vi "HFRR ADV v021 new software.vi"() -> ()   [LabVIEW 2025] (continued)
                    n2470 = Build Path(base path=w3624, name or relative path=w3626) -> (appended path=w3622:path)
                    n2471 = Number To Fractional String(number=w3652, width (-)=i16 5, precision (6)=i16 2) -> (F-format string=w3660:string)  [unwired: 1 in]
                    n2472 = local read "Fuel Discription :"() -> (w3648:string)
                    n2473 = local read "Batch Ref Num :"() -> (w3636:string)
                    n2474 = Get Date/Time String(date format (0)=enum16{"short", "long", "abbreviated"}."short") -> (date string=w3671:string, time string=w3668:string)  [unwired: 2 in]
                    n2475 = local read "Remarks :"() -> (w3647:string)
                    n2476 = Concatenate Strings("Load :- " ("Substring"), w3660, " grams ," ("Substring")) -> (w3659:string)
                    n2477 = local read "String 41"() -> (w3639:string)
                    n2478 = Concatenate Strings(w3648) -> (w3649:string)
                    n2479 = Concatenate Strings(w3636) -> (w3635:string)
                    n2480 = Concatenate Strings("tested by") -> (w3643:string)
                    n2481 = Concatenate Strings("(" ("Substring"), w3671, ")" ("Substring"), w3668) -> (w3641:string)
                    "concatenated string" <- w3641
                    n2482 = Concatenate Strings(w3647, "," ("string")) -> (w3646:string)
                    n2483 = Concatenate Strings("  TIME;      COF;       STROKE;     AIR TEMP;  TEMP;  HUMIDITY;  ECR; PID-OUT; FREQUENCY" ("Substring"), "\r") -> (w3655:string)
                    n2484 = Concatenate Strings(w3639, w3638, "Fuel Discription :-" ("Substring"), w3649, w3638, w3659, w3638, "Batch Ref Num :-" ("Substring"), w3635, w3638, " Remarks :- " ("Substring"), w3646, w3638, " Date :- " ("Substring"), w3641, w3638, "Tested By :-" ("Substring"), w3643) -> (w3653:string)
                    "REMARKS" <- w3653
                    n2485 = call <vilib>:"Write Characters To File.vi"("append to file? (new file:F)"=FALSE, "character string"=w3655, "file path (dialog if empty)"=w3623) -> ()  [unwired: 2 in, 1 out]
                    n2486 = call <vilib>:"Write Characters To File.vi"("append to file? (new file:F)"=FALSE, "character string"=w3653, "file path (dialog if empty)"=w3622) -> ()  [unwired: 2 in, 1 out]
                  }
                  frame #2 {
                    n2487 = local write "Cycles elapsed"(0 ("Cycles elapsed")) -> ()
                    n2488 = local write "cyclecount"(0 ("cyclecount")) -> ()
                    n2489 = local write "Save & Continue"(FALSE ("OK")) -> ()
                    n2490 = local write "autostrtflg"(TRUE ("autostrtflg")) -> ()
                    n2491 = local write "Save"(FALSE ("Save")) -> ()
                    n2492 = Get Date/Time In Seconds() -> (seconds since 1Jan1904=w3678:timestamp)
                    n2493 = To Double Precision Float(number=w3678) -> (double precision float=w3677:dbl)
                    n2494 = local write "acq timer"(w3677) -> ()
                    n2495 = One Button Dialog(message="Please ensure sample is mounted properly and machine is ready in all aspects for testing !", button name ("OK")="Ok") -> ()  [unwired: 1 out]
                  }
                  frame #3 {
                    n2496 = stacked-sequence {
                      frame #0 {
                        n2497 = local write "Main Dashboard Buttons"(T1."Dashboard" ("Main Dashboard Buttons")) -> ()
                        n2498 = local write "Main Tab"(T2."Acquire" ("Main Tab")) -> ()
                      }
                      frame #1 {
                        n2499 = local write "EVENT LOG"("" ("EVENT LOG")) -> ()
                      }
                      frame #2 {
                        n2500 = Wait (ms)(milliseconds to wait=u32 50) -> ()  [unwired: 1 out]
                      }
                      frame #3 {
                        n2501 = disable-structure shown="Disabled" {
                          frame Disabled {
                            n2502 = local read "EVENT LOG"() -> (w3690:string)
                            n2503 = call "Event Log.vi"("Content"="Test Details", "EVENT LOG"=w3690) -> ("EVENT LOG"=w3689:string)  [unwired: 8 in, 1 out]
                            n2504 = local write "EVENT LOG"(w3689) -> ()
                          }
                          frame Enabled {
                          }
                        }
                      }
                      frame #4 {
                        n2505 = Wait (ms)(milliseconds to wait=u32 50) -> ()  [unwired: 1 out]
                      }
                      frame #5 {
                        n2506 = local read "FILE"() -> (w3692:string)
                        n2507 = Concatenate Strings("File Name :" ("Content"), w3692) -> (w3693:string)
                        n2508 = local read "EVENT LOG"() -> (w3696:string)
                        n2509 = call "Event Log.vi"("Content"=w3693, "EVENT LOG"=w3696) -> ("EVENT LOG"=w3695:string)  [unwired: 8 in, 1 out]
                        n2510 = local write "EVENT LOG"(w3695) -> ()
                      }
                      frame #6 {
                        n2511 = Wait (ms)(milliseconds to wait=u32 50) -> ()  [unwired: 1 out]
                      }
                      frame #7 {
                        n2512 = local read "Batch Ref Num :"() -> (w3698:string)
                        n2513 = Concatenate Strings("Batch Ref No :" ("Content"), w3698) -> (w3699:string)
                        n2514 = local read "EVENT LOG"() -> (w3702:string)
                        n2515 = call "Event Log.vi"("Content"=w3699, "EVENT LOG"=w3702) -> ("EVENT LOG"=w3701:string)  [unwired: 8 in, 1 out]
                        n2516 = local write "EVENT LOG"(w3701) -> ()
                      }
                      frame #8 {
                        n2517 = Wait (ms)(milliseconds to wait=u32 50) -> ()  [unwired: 1 out]
                      }
                      frame #9 {
                        n2518 = local read "tested by"() -> (w3704:string)
                        n2519 = Concatenate Strings("Tested By :" ("Content"), w3704) -> (w3705:string)
                        n2520 = local read "EVENT LOG"() -> (w3708:string)
                        n2521 = call "Event Log.vi"("Content"=w3705, "EVENT LOG"=w3708) -> ("EVENT LOG"=w3707:string)  [unwired: 8 in, 1 out]
                        n2522 = local write "EVENT LOG"(w3707) -> ()
                      }
                      frame #10 {
                        n2523 = Wait (ms)(milliseconds to wait=u32 50) -> ()  [unwired: 1 out]
                      }
                      frame #11 {
                        n2524 = local read "TEST STANDARD"() -> (w3711:T3)
                        n2525 = case shown="\"ASTM D6079\", Default" w3711 {
                          tunnel: ["ASTM D6079" "ISO 12156" "CEC F-096-A-06" "Custom"] -> w3710
                          frame "ASTM D6079", Default {
                          }
                          frame "ISO 12156" {
                          }
                          frame "CEC F-096-A-06" {
                          }
                          frame "Custom" {
                          }
                        }
                        n2526 = Concatenate Strings("Test Standard :" ("Content"), w3710) -> (w3712:string)
                        n2527 = local read "EVENT LOG"() -> (w3715:string)
                        n2528 = call "Event Log.vi"("Content"=w3712, "EVENT LOG"=w3715) -> ("EVENT LOG"=w3714:string)  [unwired: 8 in, 1 out]
                        n2529 = local write "EVENT LOG"(w3714) -> ()
                      }
                      frame #12 {
                        n2530 = Wait (ms)(milliseconds to wait=u32 50) -> ()  [unwired: 1 out]
                      }
                      frame #13 {
                        n2531 = local read "Fuel Discription :"() -> (w3721:string)
                        n2532 = Concatenate Strings("Fuel Description :" ("Content"), w3721) -> (w3722:string)
                        n2533 = local read "EVENT LOG"() -> (w3725:string)
                        n2534 = call "Event Log.vi"("Content"=w3722, "EVENT LOG"=w3725) -> ("EVENT LOG"=w3724:string)  [unwired: 8 in, 1 out]
                        n2535 = local write "EVENT LOG"(w3724) -> ()
                      }
                      frame #14 {
                        n2536 = Wait (ms)(milliseconds to wait=u32 50) -> ()  [unwired: 1 out]
                      }
                      frame #15 {
                        n2537 = local read "Remarks :"() -> (w3727:string)
                        n2538 = Concatenate Strings("Remarks :" ("Content"), w3727) -> (w3728:string)
                        n2539 = local read "EVENT LOG"() -> (w3731:string)
                        n2540 = call "Event Log.vi"("Content"=w3728, "EVENT LOG"=w3731) -> ("EVENT LOG"=w3730:string)  [unwired: 8 in, 1 out]
                        n2541 = local write "EVENT LOG"(w3730) -> ()
                      }
                      frame #16 {
                        n2542 = Wait (ms)(milliseconds to wait=u32 50) -> ()  [unwired: 1 out]
                      }
                      frame #17 {
                        n2543 = local read "Operator ID"() -> (w3733:string)
                        n2544 = Concatenate Strings("Operator ID :" ("Content"), w3733) -> (w3735:string)
                        n2545 = local read "EVENT LOG"() -> (w3737:string)
                        n2546 = call "Event Log.vi"("Content"=w3735, "EVENT LOG"=w3737) -> ("EVENT LOG"=w3736:string)  [unwired: 8 in, 1 out]
                        n2547 = local write "EVENT LOG"(w3736) -> ()
                      }
                      frame #18 {
                        n2548 = Wait (ms)(milliseconds to wait=u32 50) -> ()  [unwired: 1 out]
                      }
                      frame #19 {
                        n2549 = disable-structure shown="Disabled" {
                          frame Disabled {
                            n2550 = local read "EVENT LOG"() -> (w3741:string)
                            n2551 = call "Event Log.vi"("Content"="Test Parameter", "EVENT LOG"=w3741) -> ("EVENT LOG"=w3740:string)  [unwired: 8 in, 1 out]
                            n2552 = local write "EVENT LOG"(w3740) -> ()
                          }
                          frame Enabled {
                          }
                        }
                      }
                      frame #20 {
                        n2553 = Wait (ms)(milliseconds to wait=u32 50) -> ()  [unwired: 1 out]
                      }
                      frame #21 {
                        n2554 = local read "Set Hz"() -> (w3745:dbl)
                        n2555 = Number To Fractional String(number=w3745, precision (6)=i16 2) -> (F-format string=w3744:string)  [unwired: 2 in]
                        n2556 = Concatenate Strings("Set Frequency [Hz] :" ("Content"), w3744) -> (w3747:string)
                        n2557 = local read "EVENT LOG"() -> (w3749:string)
                        n2558 = call "Event Log.vi"("Content"=w3747, "EVENT LOG"=w3749) -> ("EVENT LOG"=w3748:string)  [unwired: 8 in, 1 out]
                        n2559 = local write "EVENT LOG"(w3748) -> ()
                      }
                      frame #22 {
                        n2560 = Wait (ms)(milliseconds to wait=u32 50) -> ()  [unwired: 1 out]
                      }
                      frame #23 {
                        n2561 = local read "NORMAL LOAD"() -> (w3752:dbl)
                        n2562 = Number To Fractional String(number=w3752, precision (6)=i16 2) -> (F-format string=w3753:string)  [unwired: 2 in]
                        n2563 = Concatenate Strings("Applied Load [grams] :" ("Content"), w3753) -> (w3755:string)
                        n2564 = local read "EVENT LOG"() -> (w3757:string)
                        n2565 = call "Event Log.vi"("Content"=w3755, "EVENT LOG"=w3757) -> ("EVENT LOG"=w3756:string)  [unwired: 8 in, 1 out]
                        n2566 = local write "EVENT LOG"(w3756) -> ()
                      }
                      frame #24 {
                        n2567 = Wait (ms)(milliseconds to wait=u32 50) -> ()  [unwired: 1 out]
                      }
                      frame #25 {
                        n2568 = local read "Set Strk"() -> (w3760:dbl)
                        n2569 = Number To Fractional String(number=w3760, precision (6)=i16 2) -> (F-format string=w3761:string)  [unwired: 2 in]
                        n2570 = Concatenate Strings("Set Stroke [mm] :" ("Content"), w3761) -> (w3763:string)
                        n2571 = local read "EVENT LOG"() -> (w3765:string)
                        n2572 = call "Event Log.vi"("Content"=w3763, "EVENT LOG"=w3765) -> ("EVENT LOG"=w3764:string)  [unwired: 8 in, 1 out]
                        n2573 = local write "EVENT LOG"(w3764) -> ()
                      }
                      frame #26 {
                        n2574 = Wait (ms)(milliseconds to wait=u32 50) -> ()  [unwired: 1 out]
                      }
                      frame #27 {
                        n2575 = local read "Set Temp"() -> (w3768:dbl)
                        n2576 = Number To Fractional String(number=w3768, precision (6)=i16 2) -> (F-format string=w3769:string)  [unwired: 2 in]
                        n2577 = Concatenate Strings("Set Temperature [deg C] :" ("Content"), w3769) -> (w3771:string)
                        n2578 = local read "EVENT LOG"() -> (w3773:string)
                        n2579 = call "Event Log.vi"("Content"=w3771, "EVENT LOG"=w3773) -> ("EVENT LOG"=w3772:string)  [unwired: 8 in, 1 out]
                        n2580 = local write "EVENT LOG"(w3772) -> ()
                      }
                      frame #28 {
                        n2581 = Wait (ms)(milliseconds to wait=u32 50) -> ()  [unwired: 1 out]
                      }
                      frame #29 {
                        n2582 = local read "Set Rh"() -> (w3776:dbl)
                        n2583 = Number To Fractional String(number=w3776, precision (6)=i16 2) -> (F-format string=w3777:string)  [unwired: 2 in]
                        n2584 = Concatenate Strings("Set Humidity [%RH] :" ("Content"), w3777) -> (w3779:string)
                        n2585 = local read "EVENT LOG"() -> (w3781:string)
                        n2586 = call "Event Log.vi"("Content"=w3779, "EVENT LOG"=w3781) -> ("EVENT LOG"=w3780:string)  [unwired: 8 in, 1 out]
                        n2587 = local write "EVENT LOG"(w3780) -> ()
                      }
                      frame #30 {
                        n2588 = Wait (ms)(milliseconds to wait=u32 50) -> ()  [unwired: 1 out]
                      }
                      frame #31 {
                        n2589 = local read "test time"() -> (w3784:dbl)
                        n2590 = Number To Fractional String(number=w3784, precision (6)=i16 1) -> (F-format string=w3785:string)  [unwired: 2 in]
                        n2591 = Concatenate Strings("Test Duration [mins] :" ("Content"), w3785) -> (w3787:string)
                        n2592 = local read "EVENT LOG"() -> (w3789:string)
                        n2593 = call "Event Log.vi"("Content"=w3787, "EVENT LOG"=w3789) -> ("EVENT LOG"=w3788:string)  [unwired: 8 in, 1 out]
                        n2594 = local write "EVENT LOG"(w3788) -> ()
                      }
                      frame #32 {
                        w3790 = dbl[] [] ("History Data")
                        w3791 = cluster{"y":dbl, dbl, "y":dbl}[] [] ("History Data")
                        w3792 = FALSE ("Visible")
                        n2595 = property on="Stroke ( mm )" class="WFChart (strict)"("History Data"=w3791) -> ()  [unwired: 2 in, 2 out]
                        n2596 = property on="Humidity ( %RH )" class="WFChart (strict)"("History Data"=w3790) -> ()  [unwired: 2 in, 2 out]
                        n2597 = property on="Temperature ( Deg C )" class="WFChart (strict)"("History Data"=w3790) -> ()  [unwired: 2 in, 2 out]
                        n2598 = property on="Electrical Contact Resistance ( % )" class="WFChart (strict)"("History Data"=w3790) -> ()  [unwired: 2 in, 2 out]
                        n2599 = property on="Coefficient of Friction" class="WFChart (strict)"("History Data"=w3790) -> ()  [unwired: 2 in, 2 out]
                        n2600 = property on="Frictional Force ( N )" class="WFChart (strict)"("History Data"=w3790) -> ()  [unwired: 2 in, 2 out]
                        n2601 = property on="Coefficient of Friction" class="WFChart (strict)"("History Data"=w3790) -> ()  [unwired: 2 in, 2 out]
                        n2602 = property on="Frictional Force ( N )" class="WFChart (strict)"("History Data"=w3790) -> ()  [unwired: 2 in, 2 out]
                        n2603 = property on="Electrical Contact Resistance ( % )" class="WFChart (strict)"("History Data"=w3790) -> ()  [unwired: 2 in, 2 out]
                        n2604 = property on="Humidity ( %RH )" class="WFChart (strict)"("History Data"=w3790) -> ()  [unwired: 2 in, 2 out]
                        n2605 = property on="Stroke ( mm )" class="WFChart (strict)"("History Data"=w3791) -> ()  [unwired: 2 in, 2 out]
                        n2606 = property on="Temperature ( Deg C )" class="WFChart (strict)"("History Data"=w3790) -> ()  [unwired: 2 in, 2 out]
                        n2607 = property on="Service Password Log" class="Str"("Visible"=w3792) -> ()  [unwired: 2 in, 2 out]
                        n2608 = property on="Password 3" class="Clust (strict)"("Visible"=w3792) -> ()  [unwired: 2 in, 2 out]
                      }
                    }
                    "TEST FILE NAM,E SAVED" <- TRUE ("TEST FILE NAM,E SAVED")
                  }
                }
              }
            }
          }
        }
        n2609 = case shown="True" w3089 {
          frame False {
            n2610 = local write "tfalg"(0.0 ("tfalg")) -> ()
          }
          frame True {
            n2611 = local read "tfalg"() -> (w3234:dbl)
            n2612 = Equal?(x=w3234, y=0.0) -> (x = y?=w3235:bool)
            n2613 = case shown="True" w3235 {
              frame False {
              }
              frame True {
                n2614 = local read "Total No. of Tests"() -> (w3238:dbl)
                n2615 = local write "tfalg"(1.0 ("tfalg")) -> ()
                n2616 = local write "acq 2"(FALSE ("acq 2")) -> ()
                n2617 = Wait (ms)(milliseconds to wait=u32 200) -> ()  [unwired: 1 out]
                n2618 = Increment(x=w3238) -> (x+1=w3237:dbl)
                n2619 = local write "Total No. of Tests"(w3237) -> ()
              }
            }
          }
        }
        n2620 = local write "Test \nStatus"(w3095) -> ()
        n2621 = local write "Save"(w3095) -> ()
        n2622 = local read "Main Tab"() -> (w3052:T2)
        n2623 = case shown="True" w3076 {
          tunnel: [FALSE ("RUN") TRUE ("RUN")] -> w3075
          tunnel: [_ 1] -> w3068
          frame False {
          }
          frame True {
          }
        }
        n2624 = In Range and Coerce(upper limit=w3083, x=w3056, lower limit=w3082) -> (In Range?=w3074:bool)  [unwired: 1 out]
        n2625 = In Range and Coerce(upper limit=w3080, x=w3055, lower limit=w3081) -> (In Range?=w3072:bool)  [unwired: 1 out]
        n2626 = case shown="True" w3088 {
          frame False {
            n2627 = local read "Rt 3"() -> (w3216:bool)
            n2628 = case shown="True" w3216 {
              frame False {
              }
              frame True {
                n2629 = local write "Rt 3"(FALSE ("Rt 3")) -> ()
                n2630 = local write "Json End Flg"(TRUE ("Upld AR 2")) -> ()
              }
            }
            "Rt" <- TRUE ("Rt")
            "Rt 2" <- FALSE ("Rt")
          }
          frame True {
            n2631 = local read "Rt"() -> (w3223:bool)
            n2632 = local write "Rt 2"(TRUE ("Rt 2")) -> ()
            n2633 = case shown="True" w3223 {
              frame False {
              }
              frame True {
                w3224 = TRUE ("Upld AR 2")
                n2634 = local write "Rt"(FALSE ("Rt")) -> ()
                n2635 = local write "Upld AR"(w3224) -> ()
                n2636 = local write "Json St Flg"(w3224) -> ()
              }
            }
            "Rt 3" <- TRUE ("Rt 3")
          }
        }
        n2637 = case shown="True" w3074 {
          tunnel: [FALSE ("RUN") TRUE ("RUN")] -> w3073
          tunnel: [_ 2] -> w3067
          frame False {
          }
          frame True {
          }
        }
        n2638 = case shown="True" w3072 {
          tunnel: [FALSE ("RUN") TRUE ("RUN")] -> w3071
          tunnel: [_ 3] -> w3066
          frame False {
          }
          frame True {
          }
        }
        n2639 = case shown="\"Acquire\"" w3052 {
          tunnel: w3054 -> [_ w3285]
          frame Default {
            w3284 = 0.0 ("output")
            n2640 = local write "PID-out"(w3284) -> ()
            n2641 = local write "Frequency ( Hz )"(w3284) -> ()
          }
          frame "Acquire" {
            n2642 = stacked-sequence {
              frame #0 {
                n2643 = local read "Auto Start Test"() -> (w3287:bool)
                n2644 = case shown="True" w3287 {
                  tunnel: "RUN" -> [w3308 w3311]
                  tunnel: [w3308 w3310] -> w3288
                  frame False {
                  }
                  frame True {
                    n2645 = local read "Auto Start Temp"() -> (w3309:bool)
                    n2646 = Or(x=w3311, y=w3309) -> (x .or. y?=w3310:bool)
                  }
                }
                n2647 = local read "clk"() -> (w3307:dbl)
                n2648 = local read "Save"() -> (w3303:bool)
                n2649 = Equal?(x=w3307, y=0.0) -> (x = y?=w3304:bool)
                n2650 = And(x=w3304, y=w3303) -> (x .and. y?=w3305:bool)
                n2651 = Not(x="Engage") -> (.not. x?=w3294:bool)
                n2652 = case shown="False" w3288 {
                  tunnel: [0.0 w3334] -> w3290
                  frame False {
                    (unwired) TRUE ("Visible")
                    n2653 = local read "Auto Start Test"() -> (w3315:bool)
                    n2654 = local write "Start Time"(TRUE ("Start Time")) -> ()
                    n2655 = property on="Stroke 2" class="DigNum (strict)"("Visible"=FALSE) -> ()  [unwired: 2 in, 2 out]
                    n2656 = case shown="False" w3315 {
                      frame False {
                        n2657 = property on="Heater Button" class="Bool (strict)"("DisabledEnum"=T19."Enabled" ("Disabled")) -> ()  [unwired: 2 in, 2 out]
                        n2658 = property on="Humidity" class="Bool (strict)"("DisabledEnum"=T19."Enabled" ("Disabled")) -> ()  [unwired: 2 in, 2 out]
                      }
                      frame True {
                      }
                    }
                    n2659 = case shown="False" "TestCompFlg" {
                      frame False {
                        n2660 = local read "StartFlg"() -> (w3323:bool)
                        n2661 = case shown="True" w3323 {
                          frame False {
                          }
                          frame True {
                            n2662 = stacked-sequence {
                              frame #0 {
                                n2663 = local read "EVENT LOG"() -> (w3327:string)
                                n2664 = call "Event Log.vi"("Content"="Test was interrupted", "EVENT LOG"=w3327) -> ("EVENT LOG"=w3328:string)  [unwired: 8 in, 1 out]
                                n2665 = local write "EVENT LOG"(w3328) -> ()
                                n2666 = property on="RUN" class="Bool (strict)"("Visible"=TRUE) -> ()  [unwired: 2 in, 2 out]
                                n2667 = property on="Auto Start Test" class="Bool (strict)"("Visible"=TRUE) -> ()  [unwired: 2 in, 2 out]
                              }
                              frame #1 {
                                w3330 = FALSE ("StartFlg")
                                n2668 = property on="Heater Button" class="Bool (strict)"("Val(Sgnl)"=FALSE ("Value (Signaling)")) -> ()  [unwired: 2 in, 2 out]
                                n2669 = local write "Heater Button"(w3330) -> ()
                                n2670 = local write "StartFlg"(w3330) -> ()
                                n2671 = local write "Humidity"(w3330) -> ()
                              }
                              frame #2 {
                                n2672 = local write "Command"("VC;0" ("Command")) -> ()
                              }
                              frame #3 {
                                n2673 = Wait (ms)(milliseconds to wait=u32 1500) -> ()  [unwired: 1 out]
                              }
                              frame #4 {
                                n2674 = local write "Command"("HE;0" ("Command")) -> ()
                              }
                            }
                          }
                        }
                      }
                      frame True {
                      }
                    }
                    n2675 = local write "String 14"("Test will autostart once parameters reach the set value." ("String 14")) -> ()
                  }
                  frame True {
                    (unwired) FALSE ("Visible")
                    n2676 = property on="Stroke 2" class="DigNum (strict)"("Visible"=TRUE) -> ()  [unwired: 2 in, 2 out]
                    n2677 = property on="STOP 2" class="Bool (strict)"("Disabled"=u8 2) -> ()  [unwired: 2 in, 2 out]
                    n2678 = local write "String 14"(" Running....." ("String 14")) -> ()
                    n2679 = property on="Heater Button" class="Bool (strict)"("DisabledEnum"=T19."Disabled and Grayed Out" ("Disabled")) -> ()  [unwired: 2 in, 2 out]
                    n2680 = property on="Humidity" class="Bool (strict)"("DisabledEnum"=T19."Disabled and Grayed Out" ("Disabled")) -> ()  [unwired: 2 in, 2 out]
                    n2681 = case shown="True" "Start Time" {
                      selector: "Start Time" -> [_ w3353]
                      frame False {
                      }
                      frame True {
                        n2682 = Not(x=w3353) -> (.not. x?=w3352:bool)
                        n2683 = local write "Start Time"(w3352) -> ()
                        n2684 = local read "EVENT LOG"() -> (w3354:string)
                        n2685 = call "Event Log.vi"("Content"="Test in progress", "EVENT LOG"=w3354) -> ("EVENT LOG"=w3356:string)  [unwired: 8 in, 1 out]
                        n2686 = local write "EVENT LOG"(w3356) -> ()
                      }
                    }
                    n2687 = disable-structure shown="Enabled" {
                      disable-tunnel: [w3345 w3351] -> w3334
                      frame Disabled {
                        n2688 = local read "Set Hz"() -> (w3348:dbl)
                        n2689 = call <vilib>:"Uniform White Noise Waveform.vi"() -> ("signal out"=w3347:waveform(dbl))  [unwired: 10 in, 1 out]
                        n2690 = Random Number (0-1)() -> (number: 0 to 1=w3344:dbl)
                        n2691 = Add(x=w3348, y=w3347) -> (x+y=w3346:waveform(dbl))
                        n2692 = Multiply(x=ext 0.01 ("y"), y=w3344) -> (x*y=w3342:ext)
                        n2693 = Multiply(x=w3346, y=w3342) -> (x*y=w3345:waveform(ext))
                      }
                      frame Enabled {
                        n2694 = call-poly <vilib>:"Random Number (Range).vi"("lower bound (0)"=49.89, "upper bound (100)"=50.8) -> ("number"=w3351:dbl)  [unwired: 9 in]
                      }
                    }
                    "StartFlg" <- TRUE ("StartFlg")
                  }
                }
                n2695 = case shown="True" w3305 {
                  frame False {
                  }
                  frame True {
                    n2696 = local write "clk"(10.0 ("clk")) -> ()
                    n2697 = Get Date/Time In Seconds() -> (seconds since 1Jan1904=w3359:timestamp)
                    n2698 = To Double Precision Float(number=w3359) -> (double precision float=w3357:dbl)
                    n2699 = local write "acq timer"(w3357) -> ()
                    n2700 = local write "act save time"(w3357) -> ()
                  }
                }
                n2701 = call "Elapsed Time"("Time Target (s)"="Countdown", "Reset"=w3294) -> ("Elapsed Time (s)"=w3299:dbl, "Time has Elapsed"=w3297:bool)  [unwired: 10 in, 6 out]
                "Countdown 2" <- w3299
                n2702 = Subtract(x=w3299, y=2.0) -> (x-y=w3302:dbl)
                n2703 = Less?(x=w3302, y="Countdown") -> (x < y?=w3300:bool)
                n2704 = And(x=w3300, y=w3297) -> (x .and. y?=w3296:bool)
                n2705 = case shown="True" w3296 {
                  frame False {
                  }
                  frame True {
                    (unwired) dbl[] [] ("History Data")
                    n2706 = local write "Engage"(FALSE ("Engage")) -> ()
                    n2707 = local write "RUN"(TRUE ("RUN")) -> ()
                    n2708 = local read "Humidity ( %RH )"() -> (→"Rh Before":dbl)
                  }
                }
                n2709 = local read "Test \nStatus"() -> (w3292:bool)
                n2710 = Select(t=w3290, s=w3292, f=0.0) -> (s? t:f=w3291:dbl)
                n2711 = local write "Frequency ( Hz )"(w3291) -> ()
              }
              frame #1 {
                w3382 = 1000000.0 ("x")
                # "HC;1/0\nST;VALUE"
                # "Elapsed time\ncof\nstroke\nAir temp\nTemp\nHumidity"
                # "acq timer\n\nact save time"
                # "convert to microseconds"
                n2712 = local read "COUNT"() -> (w3365:i32)
                n2713 = local read "Rate"() -> (w3378:dbl)
                n2714 = Divide(x=w3382, y=w3378) -> (x/y=w3383:dbl)
                n2715 = Greater Or Equal?(x=w3365, y=250) -> (x >= y?=w3364:bool)
                n2716 = Get Date/Time In Seconds() -> (seconds since 1Jan1904=w3385:timestamp)
                n2717 = case shown="True" w3364 {
                  frame False {
                    n2718 = local read "COUNT"() -> (w3386:i32)
                    n2719 = Increment(x=w3386) -> (x+1=w3387:i32)
                    n2720 = local write "COUNT"(w3387) -> ()
                  }
                  frame True {
                    n2721 = local write "COUNT"(0 ("COUNT")) -> ()
                  }
                }
                n2722 = local read "Samplingtime 2"() -> (w3363:dbl)
                n2723 = local read "act save time"() -> (w3380:dbl)
                n2724 = Divide(x=w3383, y=w3382) -> (x/y=w3381:dbl)
                n2725 = To Double Precision Float(number=w3385) -> (double precision float=w3374:dbl)
                n2726 = Add(x=w3380, y=w3363) -> (x+y=w3379:dbl)
                n2727 = local read "acq timer"() -> (w3384:dbl)
                n2728 = local read "COUNT"() -> (w3367:i32)
                n2729 = Greater Or Equal?(x=w3374, y=w3379) -> (x >= y?=w3362:bool)
                n2730 = Multiply(x=w3381, y=w3367) -> (x*y=w3373:dbl)
                n2731 = Subtract(x=w3374, y=w3384) -> (x-y=w3376:dbl)
                n2732 = local read "Save"() -> (w3377:bool)
                n2733 = Add(x=w3376, y=w3373) -> (x+y=w3360:dbl)
                "Elapsed time 3" <- w3360
                n2734 = And(x=w3362, y=w3377) -> (x .and. y?=w3375:bool)
                n2735 = Divide(x=w3360, y=60.0) -> (x/y=w3371:dbl)
                n2736 = local read "Test \nStatus"() -> (w3361:bool)
                n2737 = local read "clk"() -> (w3368:dbl)
                n2738 = Equal?(x=w3368, y=10.0) -> (x = y?=w3370:bool)
                n2739 = case shown="True" w3375 {
                  tunnel: w3374 -> [_ w3498]
                  tunnel: [FALSE ("Boolean 2") TRUE ("Boolean 2")] -> _
                  frame False {
                  }
                  frame True {
                    w3452 = ";" ("Substring")
                    # "Pid out/\nFreq response value"
                    n2740 = local write "act save time"(w3498) -> ()
                    n2741 = local read "FILE"() -> (w3446:string)
                    n2742 = call "file check.vi"("file name in"=w3446) -> ("error out"=w3449:errorcluster, "file name out"=w3444:string)  [unwired: 9 in]
                    n2743 = local read "LVDT STROKE"() -> (w3441:dbl)
                    n2744 = local read "Add up Stroke"() -> (w3439:dbl)
                    n2745 = call "FILE PATH CREATION.vi"("error in"=w3449, "FILE NAME :"=w3444) -> ("FILE OUT"=w3447:path)  [unwired: 8 in, 1 out]
                    n2746 = Concatenate Strings(w3444, ".dgf" ("Substring")) -> (w3448:string)
                    n2747 = Subtract(x=w3441, y=w3439) -> (x-y=w3440:dbl)
                    n2748 = Absolute Value(x=w3440) -> (abs(x)=w3438:dbl)
                    n2749 = local read "FF 2"() -> (→"Frictional Force ( N )" →"Frictional Force ( N )":dbl)
                    n2750 = Build Path(base path=w3447, name or relative path=w3448) -> (appended path=w3443:path)
                    n2751 = local read "COF 2"() -> (w3457:dbl)
                    "cof" <- w3457
                    "Coefficient of Friction" <- w3457
                    "COF 4" <- w3457
                    "Coefficient of Friction" <- w3457
                    n2752 = local read "TEMP"() -> (w3460:dbl)
                    "Temp" <- w3460
                    "Temperature ( Deg C )" <- w3460
                    n2753 = local read "Humidity ( %RH )"() -> (w3459:dbl)
                    "Humidity ( %RH )" <- w3459
                    "Humidity ( %RH )" <- w3459
                    n2754 = local read "Frequency ( Hz )"() -> (w3466:dbl)
                    n2755 = call <vilib>:"Mean PtByPt.vi"("x"=w3438, "sample length"="STROKE FILTER") -> ("mean"=w3437:dbl)  [unwired: 2 in, 1 out]
                    n2756 = local read "Elapsed time"() -> (w3491:dbl)
                    n2757 = local read "AIR TEMP"() -> (w3464:dbl)
                    n2758 = local read "PID-out"() -> (w3469:dbl)
                    n2759 = local write "Temperature ( Deg C )"(w3460) -> ()
                    n2760 = Number To Fractional String(number=w3437, width (-)=i16 9 ("precision (6)"), precision (6)=i16 6) -> (F-format string=w3484:string)  [unwired: 1 in]
                    n2761 = Number To Fractional String(number=w3464, width (-)=i16 9 ("precision (6)"), precision (6)=i16 3) -> (F-format string=w3483:string)  [unwired: 1 in]
                    n2762 = Number To Fractional String(number=w3460, width (-)=i16 9 ("precision (6)"), precision (6)=i16 3) -> (F-format string=w3480:string)  [unwired: 1 in]
                    n2763 = Number To Fractional String(number=w3459, width (-)=i16 9 ("precision (6)"), precision (6)=i16 3) -> (F-format string=w3477:string)  [unwired: 1 in]
                    n2764 = Number To Fractional String(number=0.0, width (-)=i16 9 ("precision (6)"), precision (6)=i16 3) -> (F-format string=w3474:string)  [unwired: 1 in]
                    n2765 = Number To Fractional String(number=w3469, width (-)=i16 9 ("precision (6)"), precision (6)=i16 3) -> (F-format string=w3470:string)  [unwired: 1 in]
                    n2766 = Number To Fractional String(number=w3466, width (-)=i16 9 ("precision (6)"), precision (6)=i16 3) -> (F-format string=w3465:string)  [unwired: 1 in]
                    n2767 = Number To Fractional String(number=w3457, width (-)=i16 9 ("precision (6)"), precision (6)=i16 6) -> (F-format string=w3492:string)  [unwired: 1 in]
                    n2768 = Number To Fractional String(number=w3491, width (-)=i16 14 ("precision (6)"), precision (6)=i16 3) -> (F-format string=w3493:string)  [unwired: 1 in]
                    n2769 = Bundle("y"=1.02, "mean"=w3437, "y"=0.98) -> (w3458:cluster{"y":dbl, "mean":dbl, "y":dbl})  [unwired: 1 in]
                    n2770 = Number To Fractional String(number="Ambient Humidity :", width (-)=i16 9 ("precision (6)"), precision (6)=i16 6) -> (F-format string=w3450:string)  [unwired: 1 in]
                    n2771 = local read "RUN"() -> (w3456:bool)
                    n2772 = case shown="True" w3456 {
                      tunnel: w3458 -> [_ w3503]
                      tunnel: w3437 -> [_ w3502]
                      tunnel: w3437 -> [_ w3500]
                      tunnel: w3437 -> [_ w3501]
                      frame False {
                      }
                      frame True {
                        "Stroke ( mm )" <- w3503
                        "Stroke ( mm )" <- w3503
                        "Stroke 4" <- w3502
                        "Stroke 3" <- w3500
                        "Stroke 2" <- w3501
                        "measured_stroke" <- w3500
                      }
                    }
                    n2773 = Concatenate Strings(w3493, w3452, w3492, w3452, w3484, w3452, w3483, w3452, w3480, w3452, w3477, w3452, w3474, w3452, w3470, w3452, w3465, w3452, w3450, "\r") -> (w3490:string)
                    n2774 = call <vilib>:"Write Characters To File.vi"("append to file? (new file:F)"=TRUE, "character string"=w3490, "file path (dialog if empty)"=w3443) -> ()  [unwired: 2 in, 1 out]
                    "refresh flag" <- TRUE ("refresh flag")
                  }
                }
                n2775 = case shown="True" w3361 {
                  tunnel: w3371 -> [_ w3397]
                  tunnel: w3376 -> [_ w3407]
                  tunnel: [0.0 w3403] -> _
                  tunnel: w3370 -> [_ w3402]
                  tunnel: [0.0 w3401] -> _
                  tunnel: w3360 -> [_ w3401]
                  tunnel: w3374 -> [w3390 _]
                  frame False {
                    n2776 = local write "acq timer"(w3390) -> ()
                    n2777 = local write "Test Duration Status"(0.0 ("Test Duration Status")) -> ()
                  }
                  frame True {
                    n2778 = local read "Set Hz"() -> (w3404:dbl)
                    n2779 = local write "Elapsed time"(w3397) -> ()
                    n2780 = local read "test time"() -> (w3396:dbl)
                    n2781 = Multiply(x=w3407, y=w3404) -> (x*y=w3406:dbl)
                    n2782 = case shown="False" w3402 {
                      tunnel: w3406 -> [w3408 _]
                      tunnel: [w3408 1.0] -> w3403
                      frame False {
                        n2783 = local write "Cycles elapsed"(w3408) -> ()
                      }
                      frame True {
                      }
                    }
                    n2784 = Greater?(x=w3397, y=w3396) -> (0:w3405:bool)
                    n2785 = Subtract(x=w3396, y=w3397) -> (x-y=w3395:dbl)
                    "time" <- w3395
                    n2786 = Multiply(x=w3395, y=60.0) -> (x*y=w3394:dbl)
                    n2787 = local write "Time Remaining"(w3394) -> ()
                    n2788 = local write "Remaining Time"(w3394) -> ()
                    n2789 = case shown="True" w3405 {
                      frame False {
                      }
                      frame True {
                        n2790 = stacked-sequence {
                          frame #0 {
                            w3413 = T19."Enabled" ("Disabled")
                            w3412 = FALSE ("TEST FILE NAM,E SAVED")
                            w3414 = "" ("FILE")
                            w3415 = TRUE ("Visible")
                            n2791 = local write "Humidity"(FALSE ("Humidity")) -> ()
                            n2792 = local write "RUN"(FALSE ("OK Button 2")) -> ()
                            n2793 = local write "Heater Button"(FALSE ("Heater Button")) -> ()
                            n2794 = local write "Auto Start Test"(FALSE ("Auto Start Test")) -> ()
                            n2795 = local write "TestCompFlg"(TRUE ("StpFlg")) -> ()
                            n2796 = local read "Humidity ( %RH )"() -> (→"Rh After":dbl)
                            n2797 = property on="STOP 2" class="Bool (strict)"("Disabled"=u8 0) -> ()  [unwired: 2 in, 2 out]
                            n2798 = local read "EVENT LOG"() -> (w3420:string)
                            n2799 = call "Event Log.vi"("Content"="Test Completed", "EVENT LOG"=w3420) -> ("EVENT LOG"=w3419:string)  [unwired: 8 in, 1 out]
                            n2800 = property on="RUN" class="Bool (strict)"("Visible"=w3415) -> ()  [unwired: 2 in, 2 out]
                            n2801 = property on="Auto Start Test" class="Bool (strict)"("Visible"=w3415) -> ()  [unwired: 2 in, 2 out]
                            n2802 = local write "Batch Ref Num :"(w3414) -> ()
                            n2803 = local write "FILE"(w3414) -> ()
                            n2804 = local write "EVENT LOG"(w3419) -> ()
                            n2805 = local write "TEST FILE NAM,E SAVED"(w3412) -> ()
                            n2806 = local write "Fuel Discription :"(w3414) -> ()
                            n2807 = local write "START TEMP"(w3412) -> ()
                            n2808 = local write "Remarks :"(w3414) -> ()
                            n2809 = local write "Main Dashboard Buttons"(T1."Imaging" ("Main Dashboard Buttons")) -> ()
                            n2810 = local write "Main Tab"(T2."Adv Scar" ("Main Tab")) -> ()
                            n2811 = property on="FRICVALZ 2" class="Bool (strict)"("DisabledEnum"=w3413) -> ()  [unwired: 2 in, 2 out]
                            n2812 = property on="FRICVALZ 3" class="Bool (strict)"("DisabledEnum"=w3413) -> ()  [unwired: 2 in, 2 out]
                            n2813 = property on="FRICVALZ 4" class="Bool (strict)"("DisabledEnum"=w3413) -> ()  [unwired: 2 in, 2 out]
                          }
                          frame #1 {
                            n2814 = Wait (ms)(milliseconds to wait=u32 1500) -> ()  [unwired: 1 out]
                          }
                          frame #2 {
                            n2815 = local write "Command"("VC;0") -> ()
                          }
                          frame #3 {
                            n2816 = Wait (ms)(milliseconds to wait=u32 1500) -> ()  [unwired: 1 out]
                          }
                          frame #4 {
                            n2817 = local write "Command"("VC;0") -> ()
                          }
                          frame #5 {
                            n2818 = Wait (ms)(milliseconds to wait=u32 1500) -> ()  [unwired: 1 out]
                          }
                          frame #6 {
                            n2819 = local write "Command"("ST;0") -> ()
                          }
                          frame #7 {
                            n2820 = local write "measured_stroke"(0.0 ("measured_stroke")) -> ()
                            n2821 = Wait (ms)(milliseconds to wait=u32 1500) -> ()  [unwired: 1 out]
                          }
                          frame #8 {
                            n2822 = local write "Command"("HE;0") -> ()
                          }
                        }
                      }
                    }
                    n2823 = Divide(x=w3397, y=w3396) -> (x/y=w3400:dbl)
                    n2824 = Multiply(x=w3400, y=100.0) -> (x*y=w3398:dbl)
                    n2825 = local write "Test Duration Status"(w3398) -> ()
                  }
                }
              }
              frame #2 {
                n2826 = case shown="True" "Heater Button" {
                  tunnel: [0.0 ("output") w3526] -> w3504
                  frame False {
                    w3507 = TRUE ("tmpchk")
                    n2827 = local read "TEMP"() -> (w3508:dbl)
                    n2828 = local write "Temp ini"(w3508) -> ()
                    n2829 = local write "Reset 4"(w3507) -> ()
                    n2830 = local write "tmpchk"(w3507) -> ()
                    n2831 = local write "reinit"(TRUE ("reinit")) -> ()
                    n2832 = local write "manual temp log"(TRUE ("manual temp log")) -> ()
                  }
                  frame True {
                    # "Logic to turn off\nthe heater when \ntemp is not rising.\nTime - 60 sec\nDelta t- 5°c"
                    n2833 = local read "Temp ini"() -> (w3515:dbl)
                    n2834 = local read "Auto Start Test"() -> (w3511:bool)
                    n2835 = Less?(x=w3515, y=53.0) -> (x < y?=w3513:bool)
                    n2836 = case shown="False" w3511 {
                      frame False {
                        n2837 = local read "Set Temp"() -> (w3535:dbl)
                        n2838 = local read "TEMP"() -> (w3534:dbl)
                        n2839 = Subtract(x=w3535, y=w3534) -> (x-y=w3533:dbl)
                        n2840 = Absolute Value(x=w3533) -> (abs(x)=w3532:dbl)
                        n2841 = Less?(x=w3532, y=0.5) -> (x < y?=w3530:bool)
                        n2842 = case shown="True" w3530 {
                          tunnel: "manual temp log" -> [_ w3536]
                          frame False {
                          }
                          frame True {
                            n2843 = case shown="True" w3536 {
                              selector: w3536 -> [_ w3537]
                              frame False {
                              }
                              frame True {
                                # "#Event log"
                                n2844 = Not(x=w3537) -> (.not. x?=w3538:bool)
                                n2845 = local write "manual temp log"(w3538) -> ()
                                n2846 = local read "EVENT LOG"() -> (w3541:string)
                                n2847 = call "Event Log.vi"("Content"="Target Temperature reached", "EVENT LOG"=w3541) -> ("EVENT LOG"=w3540:string)  [unwired: 8 in, 1 out]
                                n2848 = local write "EVENT LOG"(w3540) -> ()
                              }
                            }
                          }
                        }
                      }
                      frame True {
                        n2849 = local write "manual temp log"(TRUE ("manual temp log")) -> ()
                      }
                    }
                    n2850 = And(x="tmpchk", y=w3513) -> (x .and. y?=w3516:bool)
                    n2851 = case shown="True" w3516 {
                      frame False {
                      }
                      frame True {
                        n2852 = call "Elapsed Time8"("Time Target (s)"=300.0, "Reset"="Reset 4") -> ("Time has Elapsed"=w3543:bool)  [unwired: 10 in, 7 out]
                        n2853 = flat-sequence {
                          tunnel: w3543 -> [_]
                          frame #0 {
                            n2854 = local write "Reset 4"(FALSE ("Reset 4")) -> ()
                          }
                        }
                        n2855 = case shown="True" w3543 {
                          frame False {
                          }
                          frame True {
                            n2856 = local read "Temp ini"() -> (w3550:dbl)
                            n2857 = Add(x=w3550, y=5.0) -> (x+y=w3548:dbl)
                            n2858 = local read "TEMP"() -> (w3551:dbl)
                            n2859 = Greater?(x=w3551, y=w3548) -> (0:w3549:bool)
                            n2860 = case shown="False" w3549 {
                              frame False {
                                n2861 = local write "Heater Button"(FALSE ("Heater Button")) -> ()
                              }
                              frame True {
                                n2862 = local write "tmpchk"(FALSE ("tmpchk")) -> ()
                              }
                            }
                          }
                        }
                      }
                    }
                    n2863 = local read "Set Temp"() -> (w3524:dbl)
                    n2864 = local read "TEMP"() -> (w3518:dbl)
                    n2865 = call-poly <vilib>:"PID.vi"("reinitialize? (F)"="reinit", "dt (s)"=-1.0, "process variable"=w3518, "setpoint"=w3524) -> ("output"=w3521:dbl)  [unwired: 6 in, 1 out]
                    n2866 = Subtract(x=w3524, y=w3518) -> (x-y=w3525:dbl)
                    n2867 = Add(x=w3524, y=0.5) -> (x+y=w3522:dbl)
                    n2868 = Greater Or Equal?(x=w3518, y=w3522) -> ()  [unwired: 1 out]
                    n2869 = Select(t=0.0, s=FALSE, f=w3521) -> (s? t:f=w3520:dbl)
                    "PID output" <- w3520
                    n2870 = flat-sequence {
                      tunnel: w3520 -> [w3554]
                      tunnel: [w3554] -> w3526
                      frame #0 {
                        n2871 = local write "reinit"(FALSE ("reinit")) -> ()
                      }
                    }
                    n2872 = Bundle(w3525, "output"=w3520, "TEMP"=w3518) -> ()  [unwired: 1 in, 1 out]
                  }
                }
                "PID-out" <- w3504
              }
              frame #3 {
                n2873 = local read "TEMP"() -> (w3556:dbl)
                n2874 = Greater Or Equal?(x=w3556, y="Set Temp 2") -> (x >= y?=w3561:bool)
                n2875 = case shown="True" w3561 {
                  tunnel: [FALSE TRUE] -> w3559
                  frame False {
                  }
                  frame True {
                  }
                }
                "Status 13" <- w3559
                n2876 = And(x=w3559, y="trip1 8") -> (x .and. y?=w3558:bool)
                n2877 = case shown="True" w3558 {
                  frame False {
                    n2878 = local write "Heater Trip Temp"(TRUE ("Heater Trip Temp")) -> ()
                  }
                  frame True {
                    w3564 = FALSE ("OK Button 2")
                    n2879 = case shown="True" "Heater Trip Temp" {
                      selector: "Heater Trip Temp" -> [_ w3566]
                      frame False {
                      }
                      frame True {
                        n2880 = Not(x=w3566) -> (.not. x?=w3565:bool)
                        n2881 = local read "EVENT LOG"() -> (w3569:string)
                        n2882 = local write "Heater Trip Temp"(w3565) -> ()
                        n2883 = call "Event Log.vi"("Content"="Heater Trip", "EVENT LOG"=w3569) -> ("EVENT LOG"=w3568:string)  [unwired: 8 in, 1 out]
                        n2884 = local write "EVENT LOG"(w3568) -> ()
                      }
                    }
                    n2885 = local write "RUN"(w3564) -> ()
                    n2886 = property on="Auto Start Test" class="Bool (strict)"("Value"=w3564) -> ()  [unwired: 2 in, 2 out]
                    n2887 = local write "Heater Button"(w3564) -> ()
                  }
                }
              }
            }
            n2888 = case shown="False" w3285 {
              frame False {
                n2889 = disable-structure shown="Disabled" {
                  frame Disabled {
                    n2890 = stacked-sequence {
                      frame #0 {
                        n2891 = local write "RUN"(FALSE ("OK Button 2")) -> ()
                      }
                      frame #1 {
                      }
                    }
                  }
                  frame Enabled {
                  }
                }
              }
              frame True {
              }
            }
          }
        }
        n2892 = local read "airtempflg"() -> (w3077:bool)
        n2893 = Or(x=w3077, y=w3075) -> (x .or. y?=w3078:bool)
        n2894 = Insert Into Array(array=string[] ["Air Temperature has reached set value,", "Humidity has reached set value,", "Sample Temperaturehas reached set value,", ""], index=0, new element="") -> (w3063:string[])
        n2895 = Build Array(w3068, w3067, w3066) -> (w3064:i32[])
        n2896 = disable-structure shown="Disabled" {
          disable-tunnel: w3078 -> [w3155 _]
          disable-tunnel: w3073 -> [w3154 _]
          disable-tunnel: w3071 -> [w3153 _]
          frame Disabled {
            n2897 = Compound Arithmetic op=AND(w3155, w3154, w3153) -> ()  [unwired: 1 out]
            n2898 = case shown="True" {
              selector: _ -> [_ _]
              frame False {
              }
              frame True {
                w3156 = FALSE ("autostrtflg")
                n2899 = local write "RUN"(TRUE ("RUN")) -> ()
                n2900 = local write "autostrtflg"(w3156) -> ()
                n2901 = local write "autostart"(w3156) -> ()
                n2902 = local write "String 14"(" Running....." ("String 14")) -> ()
              }
            }
          }
          frame Enabled {
          }
        }
        n2903 = for {
          tunnel: w3064 -> [w3206] mode=indexing
          tunnel: w3063 -> [w3205]
          shift-right: [w3202] -> w3062
          shift-left: "" -> [w3204]
          n2904 = Index Array(array=w3205, index=w3206) -> (element=w3203:string)
          n2905 = Concatenate Strings(w3203, w3204) -> (w3202:string)
        }
        n2906 = local write "autostart 2"(w3062) -> ()
        n2907 = local read "Reset Graph"() -> (w3051:bool)
        n2908 = case shown="True" w3051 {
          selector: w3051 -> [_ w3105]
          frame False {
          }
          frame True {
            w3119 = 0.0 ("X Scale.Range:Maximum")
            n2909 = Not(x=w3105) -> (.not. x?=w3104:bool)
            n2910 = local write "Reset Graph"(w3104) -> ()
            n2911 = property on="Electrical Contact Resistance ( % )" class="WFChart (strict)"("XScale.Maximum"=600.0 ("X Scale.Range:Maximum"), "XScale.Minimum"=0.0 ("X Scale.Range:Minimum"), "YScale.Maximum"=100.0 ("Y Scale.Range:Maximum"), "YScale.Minimum"=0.0 ("Y Scale.Range:Minimum")) -> ()  [unwired: 2 in, 2 out]
            n2912 = property on="Frictional Force ( N )" class="WFChart (strict)"("XScale.Maximum"=600.0 ("X Scale.Range:Maximum"), "XScale.Minimum"=0.0 ("X Scale.Range:Minimum"), "YScale.Maximum"=100.0 ("Y Scale.Range:Maximum"), "YScale.Minimum"=0.0 ("Y Scale.Range:Minimum")) -> ()  [unwired: 2 in, 2 out]
            n2913 = property on="Temperature ( Deg C )" class="WFChart (strict)"("XScale.Maximum"=600.0 ("X Scale.Range:Maximum"), "XScale.Minimum"=0.0 ("X Scale.Range:Minimum"), "YScale.Maximum"=100.0 ("Y Scale.Range:Maximum"), "YScale.Minimum"=0.0 ("Y Scale.Range:Minimum")) -> ()  [unwired: 2 in, 2 out]
            n2914 = property on="Humidity ( %RH )" class="WFChart (strict)"("XScale.Maximum"=600.0 ("X Scale.Range:Maximum"), "XScale.Minimum"=0.0 ("X Scale.Range:Minimum"), "YScale.Maximum"=100.0 ("Y Scale.Range:Maximum"), "YScale.Minimum"=0.0 ("Y Scale.Range:Minimum")) -> ()  [unwired: 2 in, 2 out]
            n2915 = property on="Stroke ( mm )" class="WFChart (strict)"("XScale.Maximum"=600.0 ("X Scale.Range:Maximum"), "XScale.Minimum"=0.0 ("X Scale.Range:Minimum"), "YScale.Maximum"=100.0 ("Y Scale.Range:Maximum"), "YScale.Minimum"=0.0 ("Y Scale.Range:Minimum")) -> ()  [unwired: 2 in, 2 out]
            n2916 = property on="Coefficient of Friction" class="WFChart (strict)"("XScale.Maximum"=600.0 ("X Scale.Range:Maximum"), "XScale.Minimum"=0.0 ("X Scale.Range:Minimum"), "YScale.Maximum"=100.0 ("Y Scale.Range:Maximum"), "YScale.Minimum"=0.0 ("Y Scale.Range:Minimum")) -> ()  [unwired: 2 in, 2 out]
            n2917 = property on="Electrical Contact Resistance ( % )" class="WFChart (strict)"("XScale.Minimum"=0.0 ("X Scale.Range:Minimum"), "XScale.Maximum"=600.0 ("X Scale.Range:Maximum"), "YScale.Minimum"=0.0 ("Y Scale.Range:Minimum"), "YScale.Maximum"=100.0 ("Y Scale.Range:Maximum")) -> ()  [unwired: 2 in, 2 out]
            n2918 = property on="Temperature ( Deg C )" class="WFChart (strict)"("XScale.Minimum"=0.0 ("X Scale.Range:Minimum"), "XScale.Maximum"=600.0 ("X Scale.Range:Maximum"), "YScale.Minimum"=0.0 ("Y Scale.Range:Minimum"), "YScale.Maximum"=100.0 ("Y Scale.Range:Maximum")) -> ()  [unwired: 2 in, 2 out]
            n2919 = property on="Coefficient of Friction" class="WFChart (strict)"("XScale.Minimum"=0.0 ("X Scale.Range:Minimum"), "XScale.Maximum"=600.0 ("X Scale.Range:Maximum"), "YScale.Maximum"=1.0 ("X Scale.Range:Minimum"), "YScale.Minimum"=0.0 ("X Scale.Range:Minimum")) -> ()  [unwired: 2 in, 2 out]
            n2920 = property on="Frictional Force ( N )" class="WFChart (strict)"("XScale.Maximum"=600.0 ("X Scale.Range:Maximum"), "XScale.Minimum"=w3119, "YScale.Maximum"=10.0 ("Y Scale.Range:Maximum"), "YScale.Minimum"=w3119) -> ()  [unwired: 2 in, 2 out]
            n2921 = property on="Stroke ( mm )" class="WFChart (strict)"("XScale.Maximum"=600.0 ("X Scale.Range:Maximum"), "XScale.Minimum"=0.0 ("X Scale.Range:Minimum"), "YScale.Maximum"=100.0 ("Y Scale.Range:Maximum"), "YScale.Minimum"=0.0 ("Y Scale.Range:Minimum")) -> ()  [unwired: 2 in, 2 out]
            n2922 = property on="Humidity ( %RH )" class="WFChart (strict)"("XScale.Maximum"=600.0 ("X Scale.Range:Maximum"), "XScale.Minimum"=0.0 ("X Scale.Range:Minimum"), "YScale.Maximum"=100.0 ("Y Scale.Range:Maximum"), "YScale.Minimum"=0.0 ("Y Scale.Range:Minimum")) -> ()  [unwired: 2 in, 2 out]
          }
        }
      }
      frame "Compare Files" {
        # "Elapsed time\ncof\nstroke\nAir temp\nTemp\nHumidity"
        n2923 = case shown="True" "RSTV1 2" {
          frame False {
          }
          frame True {
            n2924 = property on="Humidity ( %RH )" class="XYGraph (strict)"("Y Scale.Display Format:Precision"=u8 0 ("Y Scale.Format & Precision:Precision")) -> ()  [unwired: 2 in, 2 out]
            n2925 = property on="Humidity ( %RH )" class="XYGraph (strict)"("X Scale.Range:Minimum"=0.0, "X Scale.Range:Maximum"=75.0, "Y Scale.Range:Minimum"=48.0, "Y Scale.Range:Maximum"=58.0) -> ()  [unwired: 2 in, 2 out]
          }
        }
        n2926 = case shown="True" "RST CP 2" {
          frame False {
          }
          frame True {
            n2927 = property on="XY Graph 13" class="XYGraph (strict)"("Y Scale.Display Format:Precision"=u8 0 ("Y Scale.Format & Precision:Precision")) -> ()  [unwired: 2 in, 2 out]
            n2928 = property on="XY Graph 13" class="XYGraph (strict)"("X Scale.Range:Minimum"=0.0, "X Scale.Range:Maximum"=75.0, "Y Scale.Range:Minimum"=0.0, "Y Scale.Range:Maximum"=100.0) -> ()  [unwired: 2 in, 2 out]
          }
        }
        n2929 = case shown="True" "RST CP" {
          frame False {
          }
          frame True {
            n2930 = property on="Sample Temperature ( °C )" class="XYGraph (strict)"("Y Scale.Display Format:Precision"=u8 2 ("Y Scale.Format & Precision:Precision")) -> ()  [unwired: 2 in, 2 out]
            n2931 = property on="Sample Temperature ( °C )" class="XYGraph (strict)"("X Scale.Range:Minimum"=0.0, "X Scale.Range:Maximum"=75.0, "Y Scale.Range:Minimum"=58.0, "Y Scale.Range:Maximum"=62.0) -> ()  [unwired: 2 in, 2 out]
          }
        }
        n2932 = case shown="True" "RSTV1 3" {
          frame False {
          }
          frame True {
            n2933 = property on="Air Temperature  ( °C )" class="XYGraph (strict)"("Y Scale.Display Format:Precision"=u8 2 ("Y Scale.Format & Precision:Precision")) -> ()  [unwired: 2 in, 2 out]
            n2934 = property on="Air Temperature  ( °C )" class="XYGraph (strict)"("X Scale.Range:Minimum"=0.0 ("Y Scale.Range:Minimum"), "X Scale.Range:Maximum"=75.0 ("Y Scale.Range:Maximum"), "Y Scale.Range:Minimum"=20.0 ("X Scale.Range:Minimum"), "Y Scale.Range:Maximum"=26.0 ("X Scale.Range:Maximum")) -> ()  [unwired: 2 in, 2 out]
          }
        }
        n2935 = case shown="True" "RSTV1 4" {
          frame False {
          }
          frame True {
            n2936 = property on="Stroke ( mm )" class="XYGraph (strict)"("Y Scale.Display Format:Precision"=u8 2 ("Y Scale.Format & Precision:Precision")) -> ()  [unwired: 2 in, 2 out]
            n2937 = property on="Stroke ( mm )" class="XYGraph (strict)"("X Scale.Range:Minimum"=0.0 ("Y Scale.Range:Maximum"), "X Scale.Range:Maximum"=75.0 ("X Scale.Range:Minimum"), "Y Scale.Range:Minimum"=0.98, "Y Scale.Range:Maximum"=1.02) -> ()  [unwired: 2 in, 2 out]
          }
        }
        n2938 = case shown="True" "rstv2" {
          frame False {
          }
          frame True {
            n2939 = property on="Coefficient Of Friction" class="XYGraph (strict)"("Y Scale.Display Format:Precision"=u8 3 ("Y Scale.Format & Precision:Precision")) -> ()  [unwired: 2 in, 2 out]
            n2940 = property on="Coefficient Of Friction" class="XYGraph (strict)"("X Scale.Range:Minimum"=0.0 ("Y Scale.Range:Maximum"), "X Scale.Range:Maximum"=75.0, "Y Scale.Range:Minimum"=0.0, "Y Scale.Range:Maximum"=1.0 ("X Scale.Range:Minimum")) -> ()  [unwired: 2 in, 2 out]
          }
        }
        n2941 = case shown="True" "RST CP 3" {
          frame False {
          }
          frame True {
            n2942 = property on="Air Temp ( °C ) vs Humidity ( % RH )" class="XYGraph (strict)"("X Scale.Range:Minimum"=18.0, "X Scale.Range:Maximum"=28.0 ("X Scale.Range:Minimum"), "Y Scale.Range:Minimum"=30.0 ("X Scale.Range:Minimum"), "Y Scale.Range:Maximum"=70.0 ("X Scale.Range:Minimum")) -> ()  [unwired: 2 in, 2 out]
          }
        }
        n2943 = case shown="True" "OPEN 1" {
          frame False {
          }
          frame True {
            (unwired) 0  # existing file
            w3845 = "Choose a datalog file to open"  # prompt
            n2944 = local write "OPEN 1"(FALSE ("OPEN 1")) -> ()
            n2945 = String To Path(string="C:\\LAB-IQ\\Data\\") -> (path=w3830:path)
            n2946 = File Dialog(6:"*.dgf" ("pattern"), 7:w3845, 11:w3830) -> (0:w3828:errorcluster, 3:w3836:path)  [unwired: 4 in, 2 out]
            n2947 = Unbundle(w3828) -> ()  [unwired: 3 out]
            n2948 = Strip Path(path=w3836) -> (name=w3835:string)  [unwired: 1 out]
            n2949 = Path To String(path=w3836) -> (string=w3831:string)
            "string1" <- w3831
            n2950 = Match Pattern(string=w3835, regular expression=".dgf") -> (before substring=→"String Control":string)  [unwired: 1 in, 3 out]
            n2951 = Match Pattern(string=w3831, regular expression=".dgf" ("substring (\"\")")) -> (before substring=w3841:string)  [unwired: 1 in, 3 out]
            n2952 = Concatenate Strings(w3841, ".duf" ("Substring")) -> (w3837:string)
            n2953 = String To Path(string=w3837) -> (path=w3842:path)
